vi "Integrate Signals.vi"(8 "error in (no error)":errorcluster, 9 "Signals":dynamicdata(graph), 10 "Integration Length in Seconds (-1)":dbl=-1.0 format="%#_13g", 11 "Integration Offset in Seconds (0)":dbl) -> (0 "error out":errorcluster, 1 "Integration vs. Time":dynamicdata(graph), 2 "Average Integration Value":dbl, 3 "Integration Values":dbl[](graph))   [LabVIEW 2013, in "Breakdown Acoustics Controls.lvlib"]
uses:
  Breakdown Acoustics Controls/Breakdown Acoustics Controls.lvlib
panel:
  out "Array":waveform(dbl)[](array[waveform])
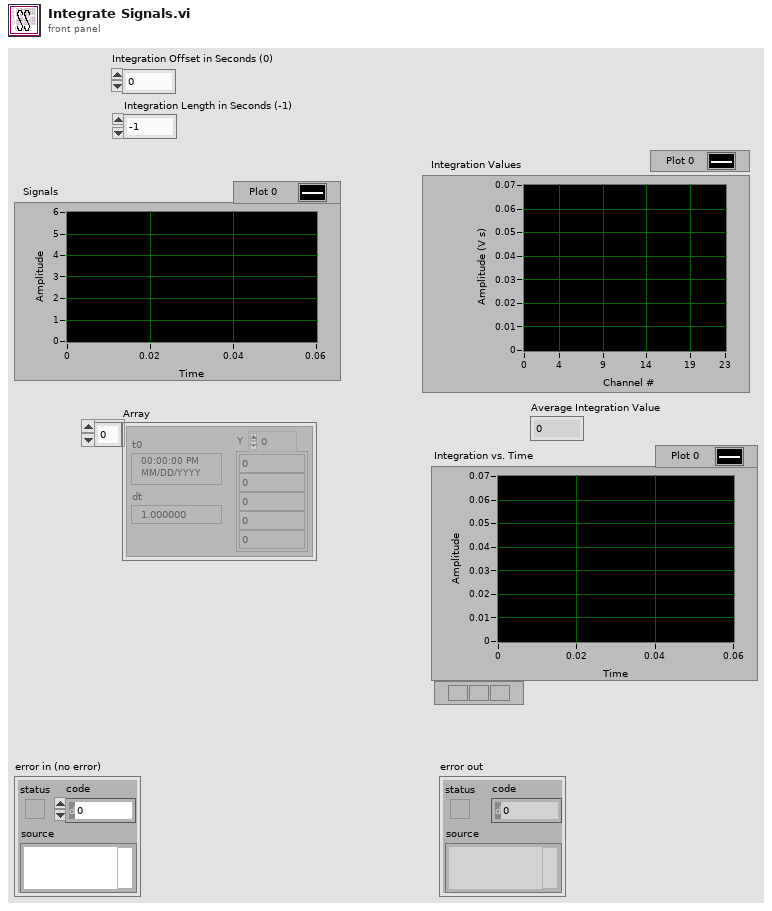
[diagram p1: front panel]
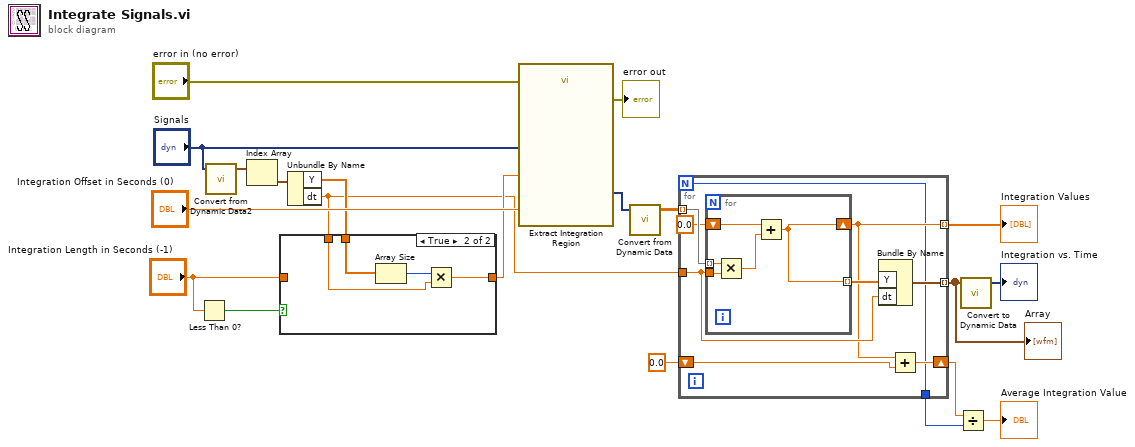
[diagram p0: block diagram]
diagram:
  n1 = Less Than 0?(x="Integration Length in Seconds (-1)") -> (x < 0?=w16:bool)
  n2 = call "Convert from Dynamic Data2"("Dynamic Data Type"="Signals") -> ("Array of Waveform"=w13:waveform(dbl)[])  [unwired: 3 in]
  n3 = Index Array(array=w13) -> (element=w10:waveform(dbl))  [unwired: 1 in]
  n4 = Unbundle By Name(w10) -> ("Y"=w11:dbl[], "dt"=w5:dbl)
  n5 = case shown="True" w16 {
    tunnel: "Integration Length in Seconds (-1)" -> [w21 _]
    tunnel: [w21 w24] -> w6
    tunnel: w5 -> [_ w23]
    tunnel: w11 -> [_ w22]
    frame False {
    }
    frame True {
      n6 = Array Size(array=w22) -> (size(s)=w25:i32)
      n7 = Multiply(x=w25, y=w23) -> (x*y=w24:dbl)
    }
  }
  n8 = call "Extract Integration Region"("error in (no error)"="error in (no error)", "Length"=w6, "Begin Offset"="Integration Offset in Seconds (0)", "Signals"="Signals") -> ("error out"=→"error out":errorcluster, "Section"=w14:dynamicdata)  [unwired: 6 in]
  n9 = call "Convert from Dynamic Data"("Dynamic Data Type"=w14) -> ("Array"=w20:dbl[][])  [unwired: 3 in]
  n10 = for {
    N -> [w26]
    tunnel: w20 -> [w34] mode=indexing
    tunnel: w5 -> [w31]
    tunnel: [w30] -> w9 mode=indexing
    tunnel: [w27] -> w8 mode=indexing
    shift-right: [w29] -> w2
    shift-left: 0.0 ("element") -> [w28]
    tunnel: [w26] -> w1
    n11 = for {
      tunnel: w34 -> [w37] mode=indexing
      shift-right: [w38] -> w27
      shift-left: 0.0 ("element") -> [w39]
      tunnel: [w38] -> w32 mode=indexing
      tunnel: w31 -> [w36]
      n12 = Multiply(x=w37, y=w36) -> (x*y=w35:dbl)
      n13 = Add(x=w39, y=w35) -> (x+y=w38:dbl)
    }
    n14 = Bundle By Name("Y"=w32, "dt"=w31) -> (w30:waveform(dbl))  [unwired: 1 in]
    n15 = Add(x=w27, y=w28) -> (x+y=w29:dbl)
  }
  "Integration Values" <- w8
  "Array" <- w9
  n16 = Divide(x=w2, y=w1) -> (x/y=→"Average Integration Value":dbl)
  n17 = call "Convert to Dynamic Data"("Array of Waveforms"=w9) -> ("Dynamic Data Type"=→"Integration vs. Time":dynamicdata)  [unwired: 3 in]
